vi "File name version detector.vi"(9 "Which file/folder?":T1, 11 "Path in":path) -> (1 "Version index (-1 = latest version)":i32, 2 "file or folder exists":bool, 3 "Path out":path)   [LabVIEW 2013]
uses:
  Typedefs/Enum-Which file or folder.ctl
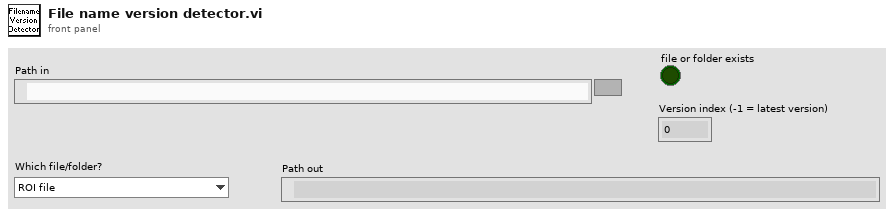
[diagram p1: front panel]
types:
  T1 = typedef "Enum-Which file or folder.ctl" = enum16{"ROI file", "Normalised ROI file", "Zplane Pockels values file", "Functional data folder"}
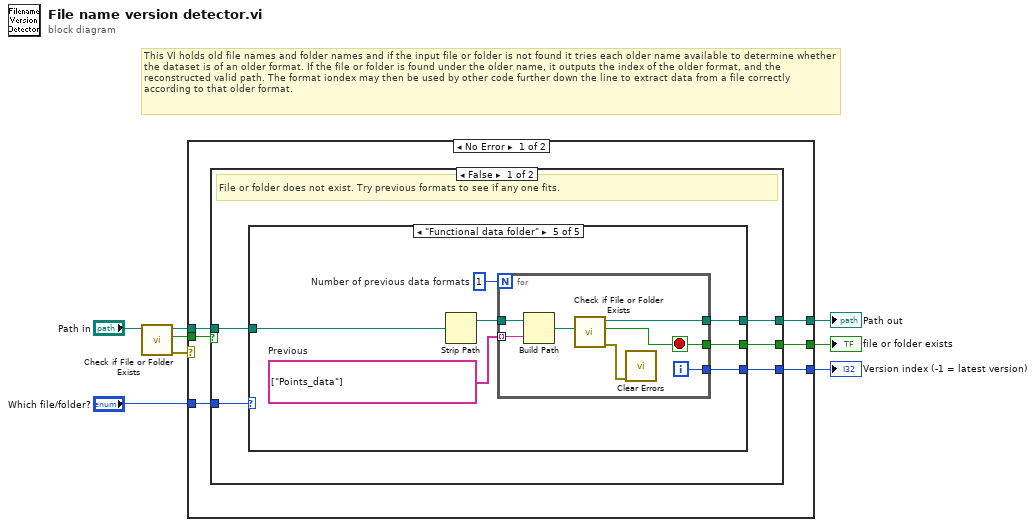
[diagram p0: block diagram]
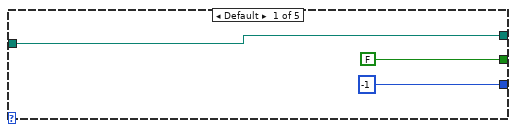
[diagram p2: hidden frame]
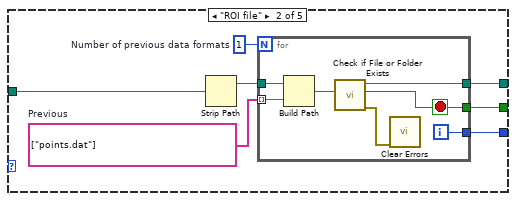
[diagram p3: hidden frame]
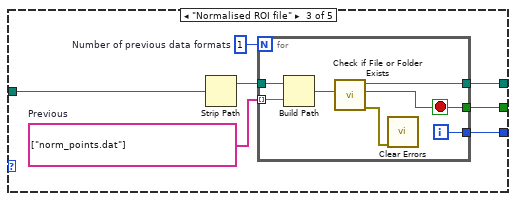
[diagram p4: hidden frame]
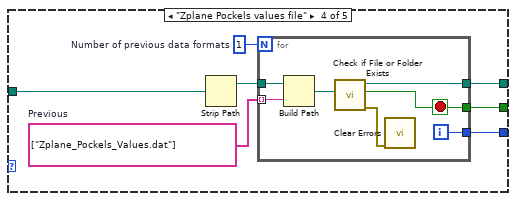
[diagram p5: hidden frame]
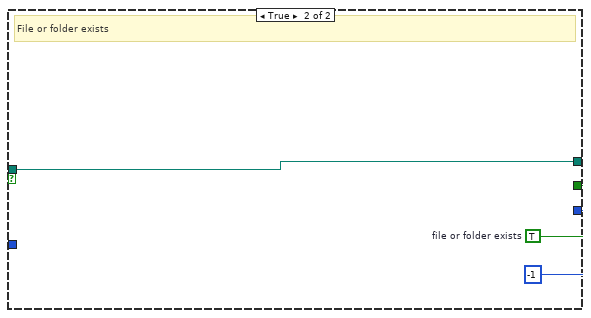
[diagram p6: hidden frame]
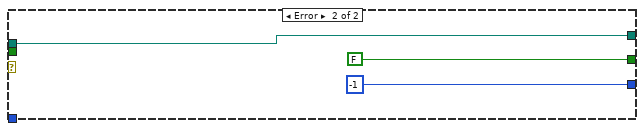
[diagram p7: hidden frame]
diagram:
  # "This VI holds old file names and folder names and if the input file or folder is not found it tries each older name available to determine whether the dataset is of an older format. If the file or folder is found under the older name, it outputs the index of the older format, and the reconstructed valid path. The format iondex may then be used by other code further down the line to extract data from a file correctly according to that older format."
  n1 = call <vilib>:"Check if File or Folder Exists.vi"("path"="Path in") -> ("error out"=w1:errorcluster, "file or folder exists?"=w7:bool, "dup path"=w6:path)  [unwired: 8 in]
  n2 = case shown="No Error" w1 {
    tunnel: w7 -> [w14 _]
    tunnel: w6 -> [w13 w84]
    tunnel: [w12 w84] -> w5
    tunnel: "Which file/folder?" -> [w11 _]
    tunnel: [w10 FALSE ("file or folder exists")] -> w3
    tunnel: [w9 -1] -> w2
    frame No Error {
      n3 = case shown="False" w14 {
        tunnel: w13 -> [w18 w81]
        tunnel: [w17 w81] -> w12
        tunnel: w11 -> [w19 _]
        tunnel: [w16 w80] -> w10
        tunnel: [w15 -1] -> w9
        frame False {
          # "File or folder does not exist. Try previous formats to see if any one fits."
          n4 = case shown="\"Functional data folder\"" w19 {
            tunnel: w18 -> [w22 w25 w39 w53 w67]
            tunnel: [w22 w29 w43 w57 w71] -> w17
            tunnel: [FALSE ("file or folder exists?") w28 w42 w56 w70] -> w16
            tunnel: [-1 w26 w40 w54 w68] -> w15
            frame Default {
            }
            frame "ROI file" {
              w23 = 1  # Number of previous data formats
              w27 = string[] ["points.dat"]  # Previous
              n5 = Strip Path(path=w25) -> (stripped path=w24:path)  [unwired: 1 out]
              n6 = for {
                N: w23 -> [_]
                tunnel: w24 -> [w36]
                tunnel: [w34] -> w29
                tunnel: [w32] -> w28
                tunnel: w27 -> [w33] mode=indexing
                tunnel: [w31] -> w26
                i -> [w31]
                stop <- w32 stop-if-true
                n7 = Build Path(base path=w36, name or relative path=w33) -> (appended path=w35:path)
                n8 = call <vilib>:"Check if File or Folder Exists.vi"("path"=w35) -> ("error out"=w30:errorcluster, "file or folder exists?"=w32:bool, "dup path"=w34:path)  [unwired: 8 in]
                n9 = call <vilib>:"Clear Errors.vi"("error in (no error)"=w30) -> ()  [unwired: 6 in, 1 out]
              }
            }
            frame "Normalised ROI file" {
              w37 = 1  # Number of previous data formats
              w41 = string[] ["norm_points.dat"]  # Previous
              n10 = Strip Path(path=w39) -> (stripped path=w38:path)  [unwired: 1 out]
              n11 = for {
                N: w37 -> [_]
                tunnel: w38 -> [w50]
                tunnel: [w48] -> w43
                tunnel: [w46] -> w42
                tunnel: w41 -> [w47] mode=indexing
                tunnel: [w45] -> w40
                i -> [w45]
                stop <- w46 stop-if-true
                n12 = Build Path(base path=w50, name or relative path=w47) -> (appended path=w49:path)
                n13 = call <vilib>:"Check if File or Folder Exists.vi"("path"=w49) -> ("error out"=w44:errorcluster, "file or folder exists?"=w46:bool, "dup path"=w48:path)  [unwired: 8 in]
                n14 = call <vilib>:"Clear Errors.vi"("error in (no error)"=w44) -> ()  [unwired: 6 in, 1 out]
              }
            }
            frame "Zplane Pockels values file" {
              w51 = 1  # Number of previous data formats
              w55 = string[] ["Zplane_Pockels_Values.dat"]  # Previous
              n15 = Strip Path(path=w53) -> (stripped path=w52:path)  [unwired: 1 out]
              n16 = for {
                N: w51 -> [_]
                tunnel: w52 -> [w64]
                tunnel: [w62] -> w57
                tunnel: [w60] -> w56
                tunnel: w55 -> [w61] mode=indexing
                tunnel: [w59] -> w54
                i -> [w59]
                stop <- w60 stop-if-true
                n17 = Build Path(base path=w64, name or relative path=w61) -> (appended path=w63:path)
                n18 = call <vilib>:"Check if File or Folder Exists.vi"("path"=w63) -> ("error out"=w58:errorcluster, "file or folder exists?"=w60:bool, "dup path"=w62:path)  [unwired: 8 in]
                n19 = call <vilib>:"Clear Errors.vi"("error in (no error)"=w58) -> ()  [unwired: 6 in, 1 out]
              }
            }
            frame "Functional data folder" {
              w65 = 1  # Number of previous data formats
              w69 = string[] ["Points_data"]  # Previous
              n20 = Strip Path(path=w67) -> (stripped path=w66:path)  [unwired: 1 out]
              n21 = for {
                N: w65 -> [_]
                tunnel: w66 -> [w78]
                tunnel: [w76] -> w71
                tunnel: [w72] -> w70
                tunnel: w69 -> [w75] mode=indexing
                tunnel: [w74] -> w68
                i -> [w74]
                stop <- w72 stop-if-true
                n22 = Build Path(base path=w78, name or relative path=w75) -> (appended path=w77:path)
                n23 = call <vilib>:"Check if File or Folder Exists.vi"("path"=w77) -> ("error out"=w73:errorcluster, "file or folder exists?"=w72:bool, "dup path"=w76:path)  [unwired: 8 in]
                n24 = call <vilib>:"Clear Errors.vi"("error in (no error)"=w73) -> ()  [unwired: 6 in, 1 out]
              }
            }
          }
        }
        frame True {
          w80 = TRUE  # file or folder exists
          # "File or folder exists"
        }
      }
    }
    frame Error {
    }
  }
  "Path out" <- w5
  "file or folder exists" <- w3
  "Version index (-1 = latest version)" <- w2
